vi "replaceCategoryUpdateConditionToken.vi"(8 "error in (no error)":errorcluster, 10 "Query In":string, 11 "Banking Transaction in":refnum<class "BankingTransaction.lvclass">) -> (0 "error out":errorcluster, 2 "Query Out":string, 3 "Banking Transaction out":refnum<class "BankingTransaction.lvclass">)   [LabVIEW 2020]
uses:
  BankingTransaction.lvclass
  Transaction/Transaction.lvclass
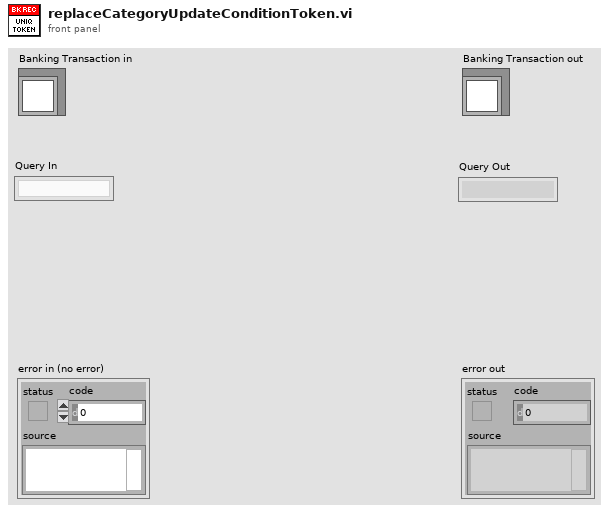
[diagram p1: front panel]
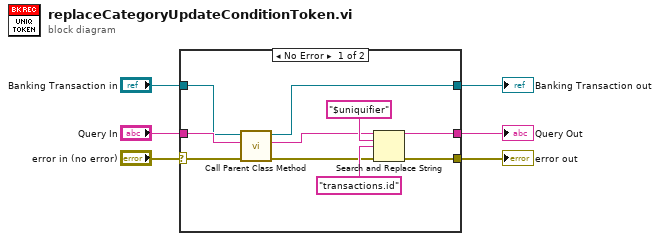
[diagram p0: block diagram]
diagram:
  n1 = case shown="No Error" "error in (no error)" {
    selector: "error in (no error)" -> [w11 w17]
    tunnel: "Query In" -> [w13 w18]
    tunnel: [w14 w18] -> w5
    tunnel: [w10 w17] -> w3
    tunnel: "Banking Transaction in" -> [w9 w19]
    tunnel: [w8 w19] -> w1
    frame No Error {
      n2 = call-parent "Call Parent Class Method"("error in (no error)"=w11, "Query In"=w13, "Transaction in"=w9) -> ("error out"=w12:errorcluster, "Query Out"=w7:string, "Transaction out"=w8:refnum<class "BankingTransaction.lvclass">)  [unwired: 6 in]
      n3 = Search and Replace String(input string=w7, search string="$uniquifier", replace string="transactions.id", error in=w12) -> (result string=w14:string, error out=w10:errorcluster)  [unwired: 4 in, 2 out]
    }
    frame Error {
    }
  }
  "error out" <- w3
  "Banking Transaction out" <- w1
  "Query Out" <- w5
